vi "cRIO_FPGA_COMMUNICATION Zähler_FGV.vi"(0 "Zählerwerte (super schneller Counter)":u16[][](array[numeric]), 1 "Zähler == 0":bool[][](array[boolean]), 2 "Set/Get/Configure":T2(ring)=enum."get Counter", 5 "Station Index":T1, 7 "Zähler":enum16{"Zähler 1", "Zähler 2", "Zähler 3"}(ring), 9 "gewünschter Zälerwert":u16, 11 "Zählerconfiguration":T3, 12 "FPGA-VI-Referenz (Ausgang)":refnum<k20>) -> (4 "ist Zähler == 0":bool[](array[boolean]), 15 "Zählerwerte":u16[](array[numeric]))   [LabVIEW 2013, in "cRIO_FPGA_COMMUNICATION.lvlib"]
uses:
  cRIO_FPGA_COMMUNICATION.lvlib
  <vilib>/rvi/interface/nirviReadWriteControl/nirviReadWriteControl.xnode
  FPGA Bitfiles/Test_FPGATarget_CScRIOPBFPGADP-M_4E0AD52E.lvbitx
  <vilib>/rvi/errors/niLvFpgaAdjustHostInterfaceError.vi
  <vilib>/rvi/errors/niLvFpgaMergeErrorWithErrorCode.vi
  NiFpgaLv.dll
  <vilib>/Utility/error.llb/Error Cluster From Error Code.vi
  TYPES/TYPE Station Index.ctl
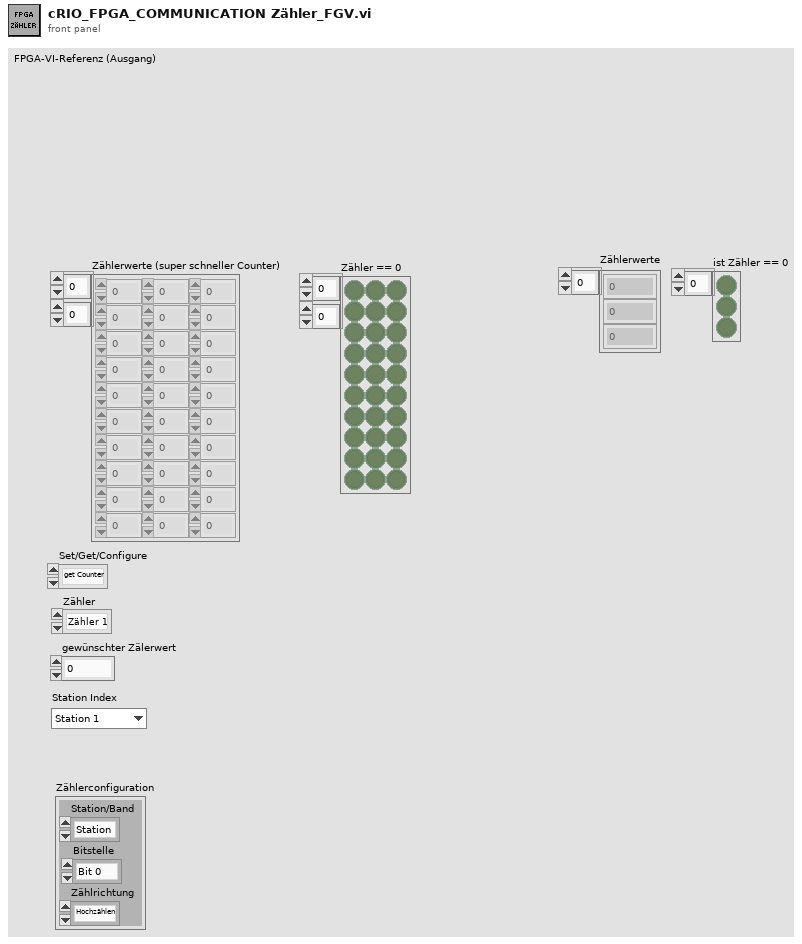
[diagram p1: front panel]
types:
  T1 = typedef "cRIO_FPGA_COMMUNICATION.lvlib/TYPE Station Index.ctl" = enum16{"Station 1", "Station 2", "Station 3", "Station 4", "Station 5", "Station 6", "Station 7", "Station 8", "Station 9", "Station 10", "Station 11", "Station 12", "Station 13", "Station 14", "Station 15", "Station 16", "Station 17", "Station 18", "Station 19", "Station 20"}
  T2 = enum16{"Init", "set Counter", "get Counter", "reset Counter", "configure Counter"}
  T3 = cluster{"Station/Band":enum16{"Station", "Band"}, "Bitstelle":enum16{"Bit 0", "Bit 1", "Bit 2", "Bit 3", "Bit 4", "Bit 5", "Bit 6", "Bit 7"}, "Zählrichtung":enum16{"Hochzählen", "Runterzählen"}}
  T4 = cluster{"Index (Station/Band)":u8, "Station/Band":enum16{"Station", "Band"}, "Bitstelle":u8, "Zählrichtung":enum16{"Hochzählen", "Runterzählen"}}[]
  T5 = cluster{"Index (Station/Band)":u8, "Station/Band":enum16{"Station", "Band"}, "Bitstelle":u8, "Zählrichtung":enum16{"Hochzählen", "Runterzählen"}}
  T6 = enum16{"Bit 0", "Bit 1", "Bit 2", "Bit 3", "Bit 4", "Bit 5", "Bit 6", "Bit 7"}
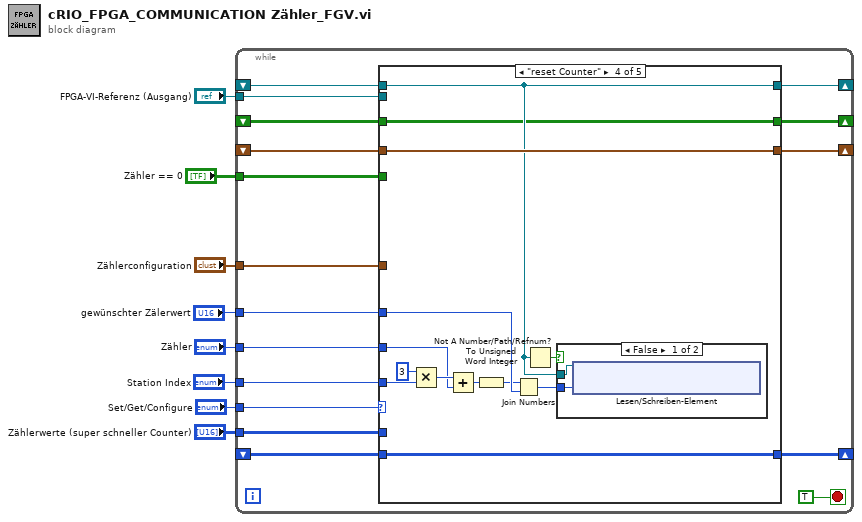
[diagram p0: block diagram]
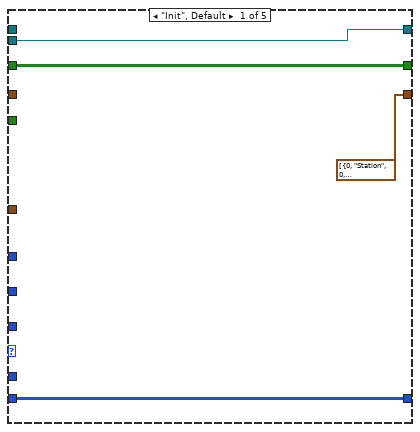
[diagram p2: hidden frame]
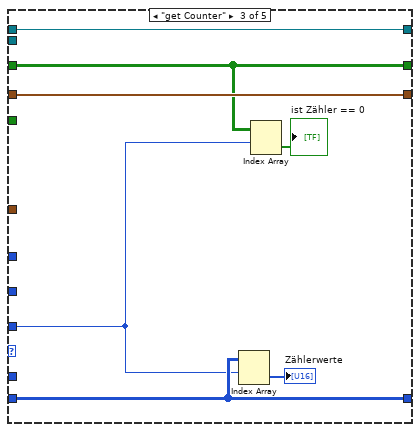
[diagram p4: hidden frame]
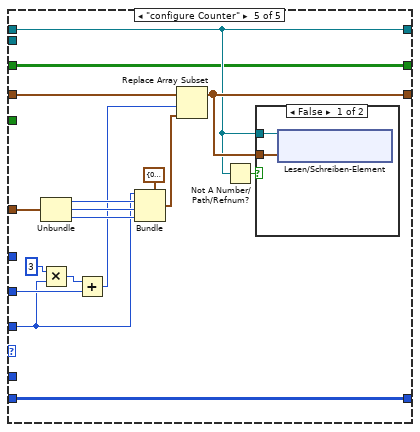
[diagram p6: hidden frame]
diagram:
  n1 = while {
    tunnel: "Zählerwerte (super schneller Counter)" -> [w22]
    tunnel: "Set/Get/Configure" -> [w24]
    tunnel: "Station Index" -> [w20]
    shift-right: [w21] -> _
    shift-left: _ -> [w23]
    tunnel: "FPGA-VI-Referenz (Ausgang)" -> [w19]
    shift-right: [w18] -> _
    shift-left: _ -> [w17]
    tunnel: "Zähler" -> [w16]
    tunnel: "gewünschter Zälerwert" -> [w15]
    tunnel: "Zählerconfiguration" -> [w12]
    shift-right: [w14] -> _
    shift-left: _ -> [w13]
    tunnel: "Zähler == 0" -> [w11]
    shift-right: [w10] -> _
    shift-left: _ -> [w9]
    stop <- TRUE stop-if-true
    n2 = case shown="\"reset Counter\"" w24 {
      tunnel: w23 -> [w29 _ w40 w53 w72]
      tunnel: [w29 w33 w40 w53 w72] -> w21
      tunnel: w22 -> [_ w33 _ _ _]
      tunnel: w20 -> [_ _ w35 w50 w59]
      tunnel: w19 -> [w28 _ _ _ _]
      tunnel: [w28 w32 w38 w42 w60] -> w18
      tunnel: w17 -> [_ w32 w38 w42 w60]
      tunnel: w16 -> [_ _ _ w49 w62]
      tunnel: w15 -> [_ _ _ w48 _]
      tunnel: [T4 [{"Index (Station/Band)"=0, "Station/Band"=enum."Station", "Bitstelle"=0, "Zählrichtung"=enum."Hochzählen"}, {"Index (Station/Band)"=0, "Station/Band"=enum."Station", "Bitstelle"=0, "Zählrichtung"=enum."Hochzählen"}, {"Index (Station/Band)"=0, "Station/Band"=enum."Station", "Bitstelle"=0, "Zählrichtung"=enum."Hochzählen"}, {"Index (Station/Band)"=0, "Station/Band"=enum."Station", "Bitstelle"=0, "Zählrichtung"=enum."Hochzählen"}, {"Index (Station/Band)"=0, "Station/Band"=enum."Station", "Bitstelle"=0, "Zählrichtung"=enum."Hochzählen"}, {"Index (Station/Band)"=0, "Station/Band"=enum."Station", "Bitstelle"=0, "Zählrichtung"=enum."Hochzählen"}, {"Index (Station/Band)"=0, "Station/Band"=enum."Station", "Bitstelle"=0, "Zählrichtung"=enum."Hochzählen"}, {"Index (Station/Band)"=0, "Station/Band"=enum."Station", "Bitstelle"=0, "Zählrichtung"=enum."Hochzählen"}, {"Index (Station/Band)"=0, "Station/Band"=enum."Station", "Bitstelle"=0, "Zählrichtung"=enum."Hochzählen"}, {"Index (Station/Band)"=0, "Station/Band"=enum."Station", "Bitstelle"=0, "Zählrichtung"=enum."Hochzählen"}, {"Index (Station/Band)"=0, "Station/Band"=enum."Station", "Bitstelle"=0, "Zählrichtung"=enum."Hochzählen"}, {"Index (Station/Band)"=0, "Station/Band"=enum."Station", "Bitstelle"=0, "Zählrichtung"=enum."Hochzählen"}, {"Index (Station/Band)"=0, "Station/Band"=enum."Station", "Bitstelle"=0, "Zählrichtung"=enum."Hochzählen"}, {"Index (Station/Band)"=0, "Station/Band"=enum."Station", "Bitstelle"=0, "Zählrichtung"=enum."Hochzählen"}, {"Index (Station/Band)"=0, "Station/Band"=enum."Station", "Bitstelle"=0, "Zählrichtung"=enum."Hochzählen"}, {"Index (Station/Band)"=0, "Station/Band"=enum."Station", "Bitstelle"=0, "Zählrichtung"=enum."Hochzählen"}, {"Index (Station/Band)"=0, "Station/Band"=enum."Station", "Bitstelle"=0, "Zählrichtung"=enum."Hochzählen"}, {"Index (Station/Band)"=0, "Station/Band"=enum."Station", "Bitstelle"=0, "Zählrichtung"=enum."Hochzählen"}, {"Index (Station/Band)"=0, "Station/Band"=enum."Station", "Bitstelle"=0, "Zählrichtung"=enum."Hochzählen"}, {"Index (Station/Band)"=0, "Station/Band"=enum."Station", "Bitstelle"=0, "Zählrichtung"=enum."Hochzählen"}, {"Index (Station/Band)"=0, "Station/Band"=enum."Station", "Bitstelle"=0, "Zählrichtung"=enum."Hochzählen"}, {"Index (Station/Band)"=0, "Station/Band"=enum."Station", "Bitstelle"=0, "Zählrichtung"=enum."Hochzählen"}, {"Index (Station/Band)"=0, "Station/Band"=enum."Station", "Bitstelle"=0, "Zählrichtung"=enum."Hochzählen"}, {"Index (Station/Band)"=0, "Station/Band"=enum."Station", "Bitstelle"=0, "Zählrichtung"=enum."Hochzählen"}, {"Index (Station/Band)"=0, "Station/Band"=enum."Station", "Bitstelle"=0, "Zählrichtung"=enum."Hochzählen"}, {"Index (Station/Band)"=0, "Station/Band"=enum."Station", "Bitstelle"=0, "Zählrichtung"=enum."Hochzählen"}, {"Index (Station/Band)"=0, "Station/Band"=enum."Station", "Bitstelle"=0, "Zählrichtung"=enum."Hochzählen"}, {"Index (Station/Band)"=0, "Station/Band"=enum."Station", "Bitstelle"=0, "Zählrichtung"=enum."Hochzählen"}, {"Index (Station/Band)"=0, "Station/Band"=enum."Station", "Bitstelle"=0, "Zählrichtung"=enum."Hochzählen"}, {"Index (Station/Band)"=0, "Station/Band"=enum."Station", "Bitstelle"=0, "Zählrichtung"=enum."Hochzählen"}] ("Zähler-Einstellung") w31 w37 w45 w69] -> w14
      tunnel: w13 -> [_ w31 w37 w45 w68]
      tunnel: w12 -> [_ _ _ _ w67]
      tunnel: w11 -> [_ w30 _ _ _]
      tunnel: [w26 w30 w36 w41 w56] -> w10
      tunnel: w9 -> [w26 _ w36 w41 w56]
      frame "Init", Default {
      }
      frame "set Counter" {
      }
      frame "get Counter" {
        n3 = Index Array(array=w40, index (row)=w35) -> (element=→"Zählerwerte":u16[])  [unwired: 1 in]
        n4 = Index Array(array=w36, index (row)=w35) -> (element=→"ist Zähler == 0":bool[])  [unwired: 1 in]
      }
      frame "reset Counter" {
        n5 = Multiply(x=3, y=w50) -> (x*y=w51:i32)
        n6 = Add(x=w51, y=w49) -> (x+y=w46:i32)
        n7 = To Unsigned Word Integer(number=w46) -> (unsigned 16bit integer=w47:u16)
        n8 = Join Numbers(hi=w47, lo=w48) -> ((hi.lo)=w43:u32)
        n9 = Not A Number/Path/Refnum?(number/path/refnum=w42) -> (NaN/Path/Refnum?=w44:bool)
        n10 = case shown="False" w44 {
          tunnel: w43 -> [w55 _]
          tunnel: w42 -> [w54 _]
          frame False {
            n11 = xnode "Lesen/Schreiben-Element"("FPGA-VI-Referenz (Eingang)"=w54, "16bitAdresen+16bitCounterwert"=w55) -> ()  [unwired: 1 in, 2 out]
          }
          frame True {
          }
        }
      }
      frame "configure Counter" {
        n12 = Unbundle(w67) -> ("Station/Band"=w66:enum16{"Station", "Band"}, "Bitstelle"=w65:T6, "Zählrichtung"=w64:enum16{"Hochzählen", "Runterzählen"})
        n13 = Multiply(x=3, y=w59) -> (x*y=w70:i32)
        n14 = Add(x=w70, y=w62) -> (x+y=w58:i32)
        n15 = Bundle(cluster=T5 {"Index (Station/Band)"=0, "Station/Band"=enum."Station", "Bitstelle"=0, "Zählrichtung"=enum."Hochzählen"} ("Cluster"), "Index (Station/Band)"=w59, "Station/Band"=w66, "Bitstelle"=w65, "Zählrichtung"=w64) -> (w63:T5)
        n16 = Replace Array Subset(array=w68, new element=w63, index=w58) -> (w69:T4)
        n17 = Not A Number/Path/Refnum?(number/path/refnum=w60) -> (NaN/Path/Refnum?=w61:bool)
        n18 = case shown="False" w61 {
          tunnel: w60 -> [w74 _]
          tunnel: w69 -> [w73 _]
          frame False {
            n19 = xnode "Lesen/Schreiben-Element"("FPGA-VI-Referenz (Eingang)"=w74, "Zähler-Einstellung"=w73) -> ()  [unwired: 1 in, 2 out]
          }
          frame True {
          }
        }
      }
    }
  }
